vi "自动复位加计数器.vi"(8 "error in":errorcluster, 9 "preset value":u32=10, 10 "reset":bool, 11 "count up":bool) -> (0 "error out":errorcluster, 1 "counter value":u32, 3 "done":bool)   [LabVIEW 2013]
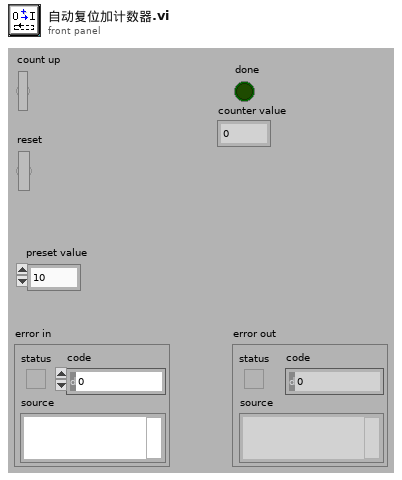
[diagram p1: front panel]
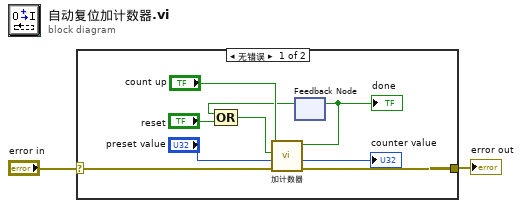
[diagram p0: block diagram]
diagram:
  n1 = case shown="无错误" "error in" {
    selector: "error in" -> [w11 w12]
    tunnel: [w10 w12] -> w2
    frame No Error {
      n2 = feedback #1() -> (w6:bool)  [unwired: 1 in]
      n3 = Compound Arithmetic op=OR(w6, "reset") -> (w4:bool)
      n4 = call "加计数器.vi"("error in"=w11, "preset value"="preset value", "reset"=w4, "count up"="count up") -> ("error out"=w10:errorcluster, "counter value"=→"counter value":u32, "done"=w7:bool)  [unwired: 5 in]
      "done" <- w7
      n5 = feedback-in #1(w7) -> ()
    }
    frame Error {
    }
  }
  "error out" <- w2
